vi "File Info__ogtk.vi"(4 "update (F)":bool, 5 "error in (no error)":errorcluster, 7 "file info":T1 {"modification date" format="%<%H:%M:%S\n%m/%d/%Y>T"; "creation date" format="%<%H:%M:%S\n%m/%d/%Y>T"; "permissions" format="%.0x"}, 8 "file":path) -> (0 "error out":errorcluster, 2 "file info":T1={"type"="????", "creator"="????", "permissions"=438, "data size"=5687, "res size"=0, "creation date"=3188231670, "modification date"=3188232972, "bFolder"=FALSE, "bInvisible"=FALSE, "location"={"vertical"=0, "horizontal"=0}, "owner"="", "group"=""} {"modification date" format="%<%H:%M:%S\n%m/%d/%Y>T"; "creation date" format="%<%H:%M:%S\n%m/%d/%Y>T"; "permissions" format="%.0x"}, 3 "file out":path)   [LabVIEW 2014]
doc: "This function either returns extended file information or changes that information for a file. For setting a particular value to something else you should first retrieve the entire information, change the value in question and write it back to disk. Be careful with this as setting wrong values for this could make the files inaccessible or even destroy it.\n\nSome of the information can be also read and modified by LabVIEW icons, others not. Following information is available in the cluster:\n\ntype: this is the Macintosh file type. This is actually also valid for the standard LabVIEW files on non-Macintosh platforms as LabVIEW stores its files in a similar fashion as what is used for Macintosh files. This value is the same as the \"type\" parameter from the Type & Creator function.\n\ntype: this is the Macintosh file creator. This is actually also valid for the standard LabVIEW files on non-Macintosh platforms as LabVIEW stores its files in a similar fashion as what is used for Macintosh files. In this case the creator is always \"LBVW\". This value is the same as the \"creator\" parameter from the Type & Creator function.\n\npermissions: This is the file access permission and is the same as is read or set with the Access Rights function.\n\ndata size: This is the same value as returned by the \"File/Directory Info\" function as well as it can be accessed by the EOF function.\n\nres size: This is the size of the Macintosh resource fork. On non Macintosh systems this value is always 0.\n\ncreation date: The creation date of the file as far as the OS file system supports that. Changing this value is under normal circumstances probably not a good idea. For instance making this date to be later than the modification date could cause certain issues on some systems.\n\nmodification date: This value is the same as returned by the \"File/Directory Info\" LabVIEW node.\n\nbFolder: If non-zero indicates that the path points to a directory. This value is the same as returned by the \"File/Directory Info\" function.\n\nbInvisible: If non-zero indicates if the file has the OS dependant hidden flag set.\n\nlocation: System specific desktop geographical location (on Mac only)"
uses:
  File Info Record__ogtk.ctl
panel:
  # "File Info.vi\n\nSets or reads the information for a file.\n\nPlease visit http://www.OpenG.org to learn about the\nOpen Source LabVIEW software movement.\n\nNOTICE -- YOU MUST LEAVE THIS NOTICE IN PLACE.  PER THE TERMS OF THE LICENSE BELOW, YOU MAY SUBLICENSE THIS SOFTWARE \nIN ANY WAY THAT DOES NOT CONFLICT WITH THIS LICENSE.\n\n### BSD License (http://www.opensource.org/licenses/bsd-license.php) Begin ###\n\nCopyright (c) 2002-2005, Rolf Kalbermatter <rolf.kalbermatter@citeng.com>\nCopyright (c) 2006, Jim Kring <jim@jimkring.com>\n\nAll rights reserved.\n\nRedistribution and use in source and binary forms, with or without modification, are permitted provided that the following conditions are met:\n\n    * Redistributions of source code must retain the above copyright notice, this list of conditions and the following disclaimer.\n    * Redistributions in binary form must reproduce the above copyright notice, this list of conditions and the following disclaimer in the \n       documentation and/or other materials provided with the distribution.\n    * Neither the name of SciWare, James Kring, Inc., nor the names of its contributors may be used to endorse or promote products derived \n       from this software without specific prior written permission.\n\nTHIS SOFTWARE IS PROVIDED BY THE COPYRIGHT HOLDERS AND CONTRIBUTORS \"AS IS\" AND ANY EXPRESS OR IMPLIED WARRANTIES, \nINCLUDING, BUT NOT LIMITED TO, THE IMPLIED WARRANTIES OF MERCHANTABILITY AND FITNESS FOR A PARTICULAR PURPOSE ARE \nDISCLAIMED. IN NO EVENT SHALL THE COPYRIGHT OWNER OR CONTRIBUTORS BE LIABLE FOR ANY DIRECT, INDIRECT, INCIDENTAL,\n SPECIAL, EXEMPLARY, OR CONSEQUENTIAL DAMAGES (INCLUDING, BUT NOT LIMITED TO, PROCUREMENT OF SUBSTITUTE GOODS OR \nSERVICES; LOSS OF USE, DATA, OR PROFITS; OR BUSINESS INTERRUPTION) HOWEVER CAUSED AND ON ANY THEORY OF LIABILITY, \nWHETHER IN CONTRACT, STRICT LIABILITY, OR TORT (INCLUDING NEGLIGENCE OR OTHERWISE) ARISING IN ANY WAY OUT OF THE USE \nOF THIS SOFTWARE, EVEN IF ADVISED OF THE POSSIBILITY OF SUCH DAMAGE.\n\n### BSD License End ###"
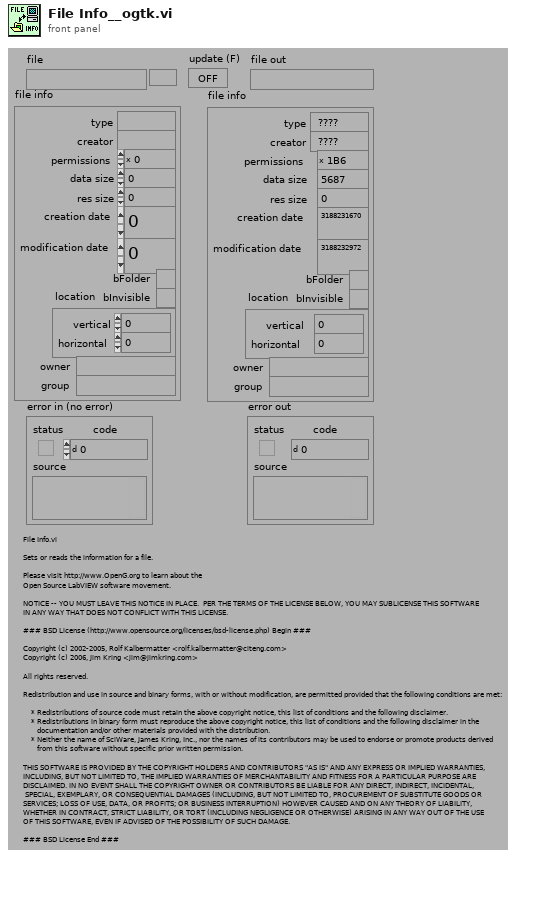
[diagram p1: front panel]
types:
  T1 = typedef "File Info Record__ogtk.ctl" = cluster{"type":string, "creator":string, "permissions":i32, "data size":i32, "res size":i32, "creation date":u32, "modification date":u32, "bFolder":bool, "bInvisible":bool, "location":cluster{"vertical":i16, "horizontal":i16}, "owner":string, "group":string}
  T2 = cluster{"permissions":i32, "data size":i32, "res size":i32, "creation date":u32, "modification date":u32, "bFolder":i32, "bInvisible":i32, "location":cluster{"vertical":i16, "horizontal":i16}}
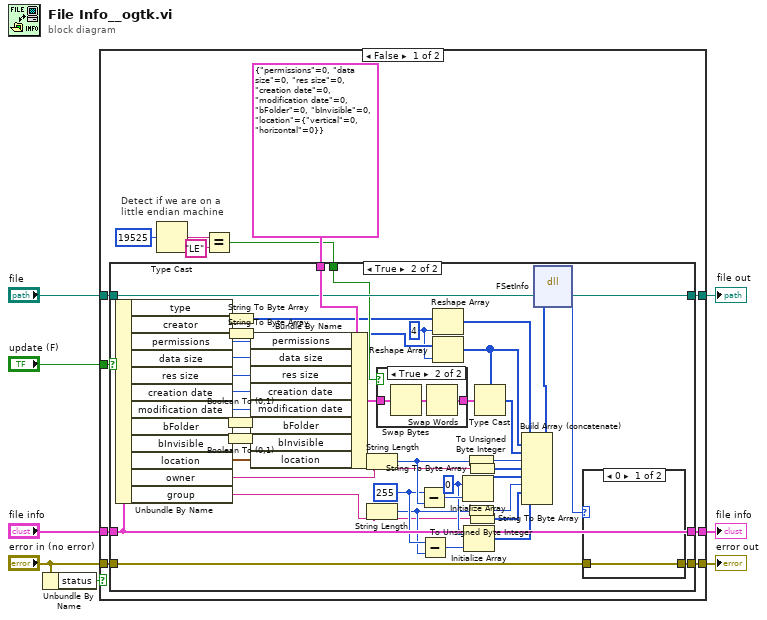
[diagram p0: block diagram]
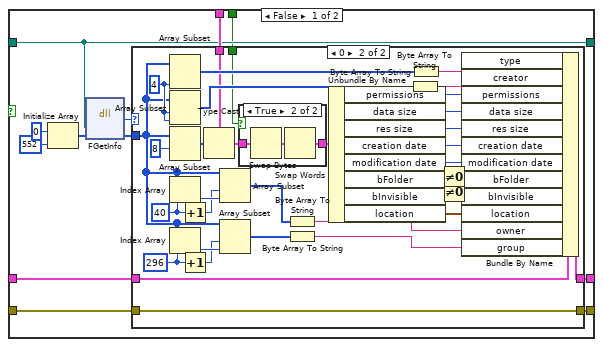
[diagram p2: hidden frame]
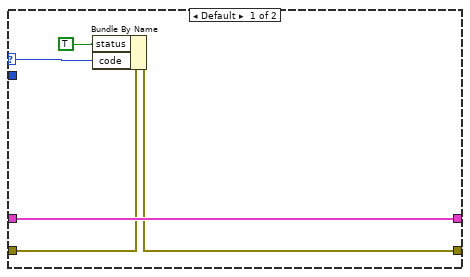
[diagram p3: hidden frame]
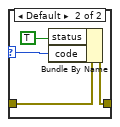
[diagram p6: hidden frame]
diagram:
  n1 = Unbundle By Name("error in (no error)") -> ("status"=w2:bool)
  n2 = case shown="False" w2 {
    tunnel: "error in (no error)" -> [w20 w130]
    tunnel: [w19 w130] -> w7
    tunnel: [w18 w131] -> w6
    tunnel: "file info" -> [w17 w131]
    tunnel: "file" -> [w15 w129]
    tunnel: [w14 w129] -> w3
    tunnel: "update (F)" -> [w13 _]
    frame False {
      # "Detect if we are on a\nlittle endian machine"
      n3 = Type Cast(x=i16 19525) -> (*(type *) &x=w11:string)  [unwired: 1 in]
      n4 = Equal?(x=w11, y="LE") -> (x = y?=w12:bool)
      n5 = case shown="True" w13 {
        tunnel: w20 -> [w25 w101]
        tunnel: [w24 w100] -> w19
        tunnel: [w27 w104] -> w18
        tunnel: w17 -> [w28 w104]
        tunnel: T2 {"permissions"=0, "data size"=0, "res size"=0, "creation date"=0, "modification date"=0, "bFolder"=0, "bInvisible"=0, "location"={"vertical"=0, "horizontal"=0}} -> [w29 w119]
        tunnel: w15 -> [w23 w105]
        tunnel: [w23 w103] -> w14
        tunnel: w12 -> [w22 w99]
        frame False {
          n6 = Initialize Array(u8 0 ("Element Data"), 552 ("Dimension Size")) -> (w31:u8[])
          n7 = dll-call lib="LabVIEW" fn="FGetInfo"("file"=w23, "infop"=w31) -> (w26:i32, "infop"=w21:u8[])  [unwired: 4 in, 2 out]
          n8 = case shown="0" w26 {
            selector: w26 -> [w33 _]
            tunnel: w21 -> [_ w40]
            tunnel: w29 -> [_ w68]
            tunnel: w28 -> [w37 w66]
            tunnel: [w37 w65] -> w27
            tunnel: w25 -> [w36 w53]
            tunnel: [w35 w53] -> w24
            tunnel: w22 -> [_ w52]
            frame Default {
              n9 = Bundle By Name(cluster=w36, "status"=TRUE, "code"=w33) -> (w35:errorcluster)
            }
            frame 0 {
              w41 = 296 ("index")
              w47 = 40 ("index")
              w72 = 4 ("Array Length")
              n10 = Array Subset(array=w40, length=w72) -> (w70:u8[])  [unwired: 1 in]
              n11 = Array Subset(array=w40, index=w72, length=w72) -> (w69:u8[])
              n12 = Array Subset(array=w40, index=8 ("Array Index")) -> (w49:u8[])  [unwired: 1 in]
              n13 = Index Array(array=w40, index=w47) -> (element=w48:u8)
              n14 = Index Array(array=w40, index=w41) -> (element=w43:u8)
              n15 = Increment(x=w47) -> (x+1=w46:i32)
              n16 = Increment(x=w41) -> (x+1=w42:i32)
              n17 = Type Cast(type=w68, x=w49) -> (*(type *) &x=w67:T2)
              n18 = Array Subset(array=w40, index=w46, length=w48) -> (w45:u8[])
              n19 = Array Subset(array=w40, index=w42, length=w43) -> (w39:u8[])
              n20 = case shown="True" w52 {
                tunnel: w67 -> [w73 w76]
                tunnel: [w73 w74] -> w64
                frame False {
                }
                frame True {
                  n21 = Swap Bytes(anything=w76) -> (byte swapped=w75:T2)
                  n22 = Swap Words(1:w75) -> (0:w74:T2)
                }
              }
              n23 = Byte Array To String(unsigned byte array=w45) -> (string=w44:string)
              n24 = Byte Array To String(unsigned byte array=w39) -> (string=w38:string)
              n25 = Unbundle By Name(w64) -> ("permissions"=w56:i32, "data size"=w57:i32, "res size"=w58:i32, "creation date"=w59:u32, "modification date"=w60:u32, "bFolder"=w61:i32, "bInvisible"=w62:i32, "location"=w63:cluster{"vertical":i16, "horizontal":i16})
              n26 = Byte Array To String(unsigned byte array=w69) -> (string=w55:string)
              n27 = Byte Array To String(unsigned byte array=w70) -> (string=w54:string)
              n28 = Not Equal To 0?(x=w61) -> (x != 0?=w51:bool)
              n29 = Not Equal To 0?(x=w62) -> (x != 0?=w50:bool)
              n30 = Bundle By Name(cluster=w66, "type"=w54, "creator"=w55, "permissions"=w56, "data size"=w57, "res size"=w58, "creation date"=w59, "modification date"=w60, "bFolder"=w51, "bInvisible"=w50, "location"=w63, "owner"=w44, "group"=w38) -> (w65:T1)
            }
          }
        }
        frame True {
          w81 = u8 0 ("Element Data")
          w80 = 255
          w92 = 4 ("Dimension Size")
          n31 = Unbundle By Name(w104) -> ("type"=w109:string, "creator"=w110:string, "permissions"=w111:i32, "data size"=w112:i32, "res size"=w113:i32, "creation date"=w114:u32, "modification date"=w115:u32, "bFolder"=w116:bool, "bInvisible"=w117:bool, "location"=w118:cluster{"vertical":i16, "horizontal":i16}, "owner"=w86:string, "group"=w77:string)
          n32 = Boolean To (0,1)(Boolean=w116) -> (0, 1=w97:i16)
          n33 = Boolean To (0,1)(Boolean=w117) -> (0, 1=w96:i16)
          n34 = String To Byte Array(string=w109) -> (unsigned byte array=w95:u8[])
          n35 = String To Byte Array(string=w110) -> (unsigned byte array=w93:u8[])
          n36 = Bundle By Name(cluster=w119, "permissions"=w111, "data size"=w112, "res size"=w113, "creation date"=w114, "modification date"=w115, "bFolder"=w97, "bInvisible"=w96, "location"=w118) -> (w98:T2)
          n37 = String Length(string=w86) -> (length=w106:i32)
          n38 = String Length(string=w77) -> (length=w78:i32)
          n39 = case shown="True" w99 {
            tunnel: w98 -> [w120 w123]
            tunnel: [w120 w121] -> w108
            frame False {
            }
            frame True {
              n40 = Swap Bytes(anything=w123) -> (byte swapped=w122:T2)
              n41 = Swap Words(1:w122) -> (0:w121:T2)
            }
          }
          n42 = Subtract(x=w80, y=w106) -> (x-y=w89:i32)
          n43 = Subtract(x=w80, y=w78) -> (x-y=w79:i32)
          n44 = Reshape Array(w95, w92) -> (w94:u8[])
          n45 = Reshape Array(w93, w92) -> (w90:u8[])
          n46 = Initialize Array(w81, w89) -> (w85:u8[])
          n47 = Initialize Array(w81, w79) -> (w82:u8[])
          n48 = To Unsigned Byte Integer(number=w106) -> (unsigned 8bit integer=w87:u8)
          n49 = To Unsigned Byte Integer(number=w78) -> (unsigned 8bit integer=w84:u8)
          n50 = String To Byte Array(string=w86) -> (unsigned byte array=w88:u8[])
          n51 = String To Byte Array(string=w77) -> (unsigned byte array=w83:u8[])
          n52 = Type Cast(type=w90, x=w108) -> (*(type *) &x=w107:u8[])
          n53 = Build Array (concatenate)(w94, w90, w107, w87, w88, w85, w84, w83, w82) -> (w91:u8[])
          n54 = dll-call lib="LabVIEW" fn="FSetInfo"("file"=w105, "infop"=w91) -> (w102:i32, "file"=w103:path)  [unwired: 4 in, 2 out]
          n55 = case shown="0" w102 {
            selector: w102 -> [_ w127]
            tunnel: w101 -> [w124 w126]
            tunnel: [w124 w125] -> w100
            frame 0 {
            }
            frame Default {
              n56 = Bundle By Name(cluster=w126, "status"=TRUE, "code"=w127) -> (w125:errorcluster)
            }
          }
        }
      }
    }
    frame True {
    }
  }
  "error out" <- w7
  "file info" <- w6
  "file out" <- w3
